vi "CalculateTresholdForPeakDetection.vi"(11 "Array":dbl[](array[numeric])) -> (3 "Average":dbl)   [LabVIEW 2013]
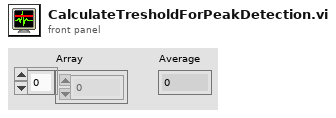
[diagram p1: front panel]
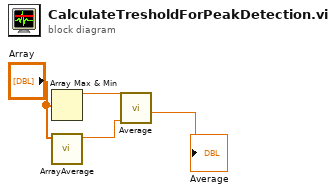
[diagram p0: block diagram]
diagram:
  n1 = Array Max & Min(array="Array") -> (max value=w2:dbl)  [unwired: 3 out]
  n2 = call "ArrayAverage.vi"("array"="Array") -> ("Average"=w3:dbl)  [unwired: 10 in]
  n3 = call "Average.vi"("y"=w3, "x"=w2) -> ("Average"=→"Average":dbl)  [unwired: 9 in]
